vi "Add Pattern Part.vi"(4 "Suffix":string, 6 "Prefix":string, 8 "Modifier Token":T1, 9 "Regexp or Wildcard Token":T1, 10 "Name Token":T1, 11 "Pattern Parser In":T3) -> (0 "error out":errorcluster, 3 "Pattern Parser":T3)   [LabVIEW 2020, in "Stream.lvlib" / "URLPattern.lvclass"]
uses:
  URLPattern.lvclass
  Pattern Part Modifier.ctl
  Pattern Part Type.ctl
  Pattern Part.ctl
  Token Type.ctl
  Token.ctl
  Pattern Parser.ctl
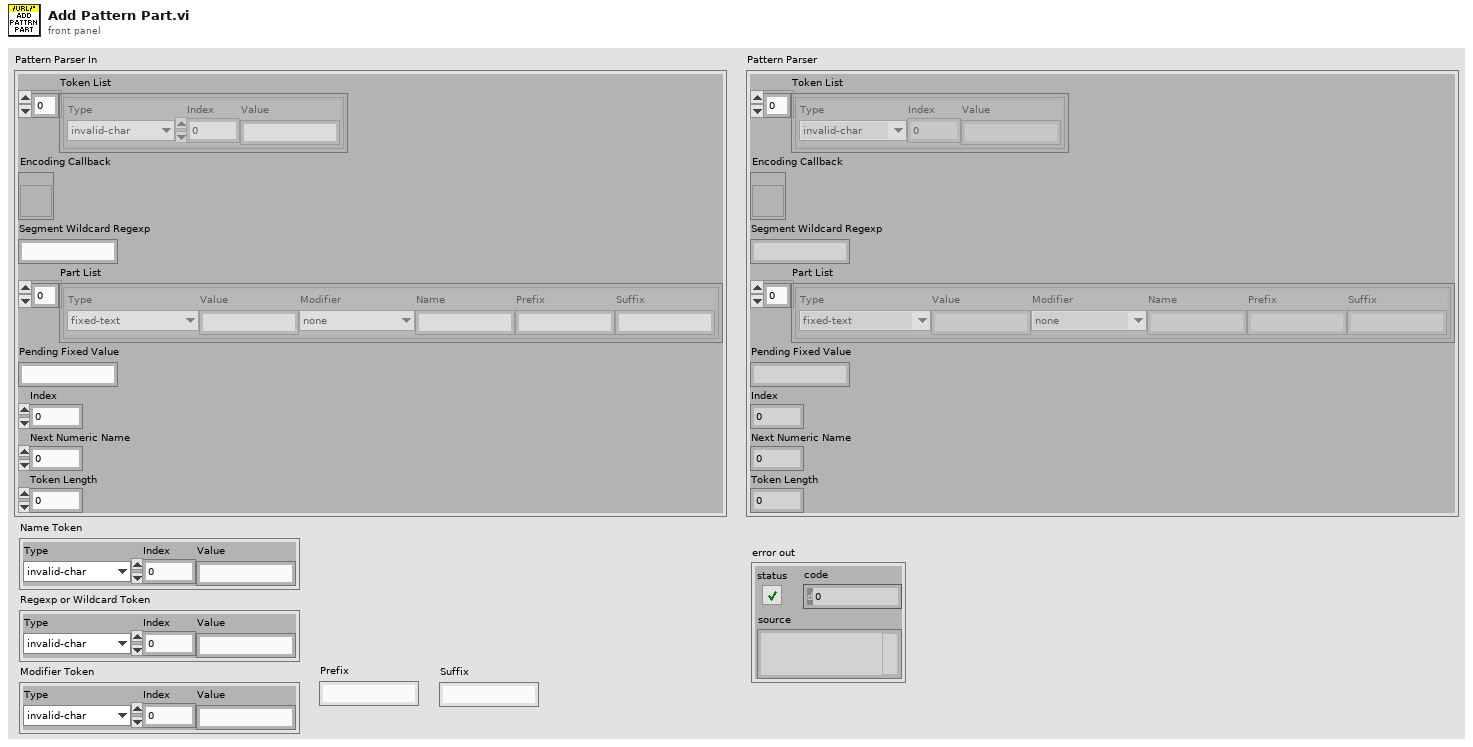
[diagram p1: front panel]
types:
  T1 = typedef "Stream.lvlib/URLPattern.lvclass/Token.ctl" = cluster{"Type":T2, "Index":i32, "Value":string}
  T2 = typedef "Stream.lvlib/URLPattern.lvclass/Token Type.ctl" = enum16{"invalid-char", "open", "close", "regexp", "name", "char", "escaped-char", "other-modifier", "asterisk", "end"}
  T3 = typedef "Stream.lvlib/URLPattern.lvclass/Pattern Parser.ctl" = cluster{"Token List":T1[], "Encoding Callback":refnum<vi>, "Segment Wildcard Regexp":string, "Part List":T4[], "Pending Fixed Value":string, "Index":i32, "Next Numeric Name":i32, "Token Length":i32}
  T4 = typedef "Stream.lvlib/URLPattern.lvclass/Pattern Part.ctl" = cluster{"Type":T5, "Value":string, "Modifier":T6, "Name":string, "Prefix":string, "Suffix":string}
  T5 = typedef "Stream.lvlib/URLPattern.lvclass/Pattern Part Type.ctl" = enum16{"fixed-text", "regexp", "segment-wildcard", "full-wildcard"}
  T6 = typedef "Stream.lvlib/URLPattern.lvclass/Pattern Part Modifier.ctl" = enum16{"none", "optional", "zero-or-more", "one-or-more"}
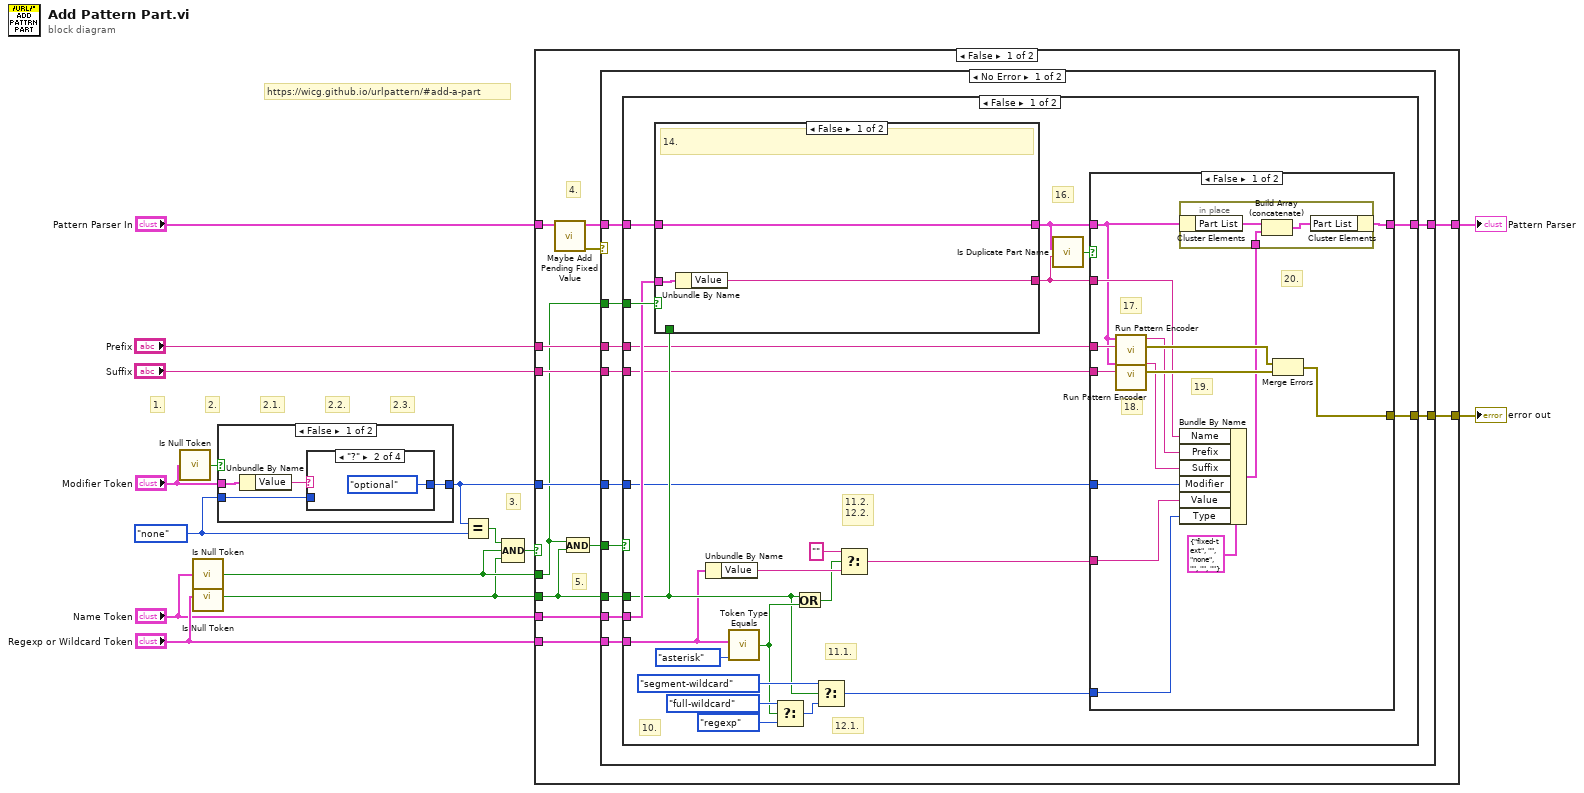
[diagram p0: block diagram]
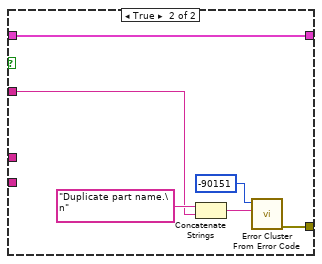
[diagram p2: hidden frame]
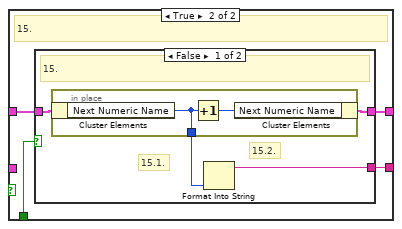
[diagram p3: hidden frame]
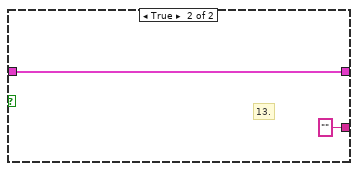
[diagram p4: hidden frame]
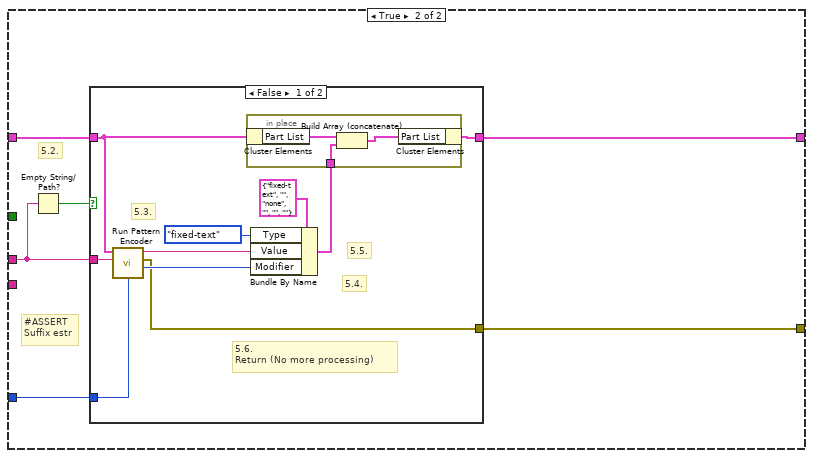
[diagram p5: hidden frame]
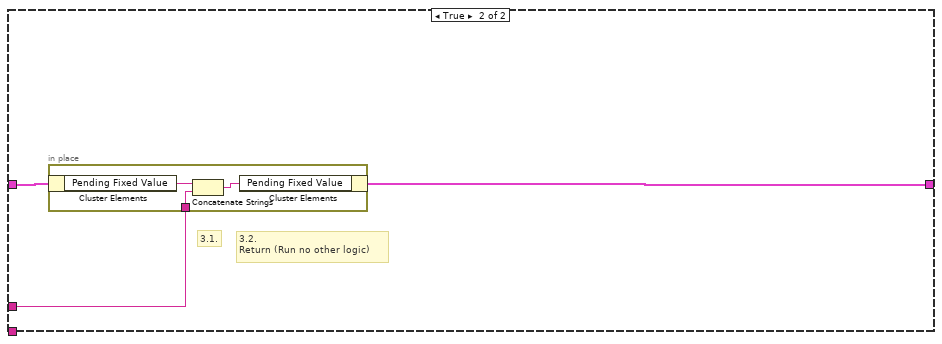
[diagram p8: hidden frame]
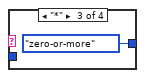
[diagram p10: hidden frame]
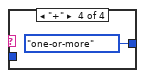
[diagram p11: hidden frame]
diagram:
  w7 = Pattern_Part_Modifier."none" ("Pattern Part Modifier")
  # "3."
  # "2.3."
  # "2.2."
  # "2.1."
  # "2."
  # "1."
  # "https://wicg.github.io/urlpattern/#add-a-part"
  n1 = call "Is Null Token.vi"("Token"="Modifier Token") -> ("Null Token"=w15:bool)
  n2 = call "Is Null Token.vi"("Token"="Name Token") -> ("Null Token"=w5:bool)
  n3 = call "Is Null Token.vi"("Token"="Regexp or Wildcard Token") -> ("Null Token"=w4:bool)
  n4 = case shown="False" w15 {
    tunnel: "Modifier Token" -> [w19 _]
    tunnel: [w17 w24] -> w6
    tunnel: w7 -> [w16 w24]
    frame False {
      n5 = Unbundle By Name(w19) -> ("Value"=w18:string)
      n6 = case shown="\"?\"" w18 {
        tunnel: [w20 Pattern_Part_Modifier."optional" ("Pattern Part Modifier") Pattern_Part_Modifier."zero-or-more" ("Pattern Part Modifier") Pattern_Part_Modifier."one-or-more" ("Pattern Part Modifier")] -> w17
        tunnel: w16 -> [w20 _ _ _]
        frame Default {
        }
        frame "?" {
        }
        frame "*" {
        }
        frame "+" {
        }
      }
    }
    frame True {
    }
  }
  n7 = Equal?(x=w6, y=w7) -> (x = y?=w13:bool)
  n8 = Compound Arithmetic op=AND(w13, w5, w4) -> (w12:bool)
  n9 = case shown="False" w12 {
    tunnel: "Pattern Parser In" -> [w37 w135]
    tunnel: "Prefix" -> [w33 w134]
    tunnel: [w32 w133] -> w9
    tunnel: "Suffix" -> [w35 _]
    tunnel: w6 -> [w31 _]
    tunnel: w5 -> [w28 _]
    tunnel: w4 -> [w29 _]
    tunnel: "Regexp or Wildcard Token" -> [w30 _]
    tunnel: "Name Token" -> [w27 _]
    tunnel: [w26 _] -> w1
    frame False {
      # "5."
      # "4."
      n10 = call "Maybe Add Pending Fixed Value.vi"("Pattern Parser In"=w37) -> ("error out"=w25:errorcluster, "Pattern Parser"=w36:T3)  [unwired: 9 in]
      n11 = And(x=w28, y=w29) -> (x .and. y?=w34:bool)
      n12 = case shown="No Error" w25 {
        selector: w25 -> [_ w132]
        tunnel: w36 -> [w48 w131]
        tunnel: w35 -> [w47 _]
        tunnel: w34 -> [w46 _]
        tunnel: w33 -> [w45 _]
        tunnel: [w44 w131] -> w32
        tunnel: w31 -> [w43 _]
        tunnel: w30 -> [w42 _]
        tunnel: w29 -> [w41 _]
        tunnel: w28 -> [w40 _]
        tunnel: w27 -> [w39 _]
        tunnel: [w38 w132] -> w26
        frame No Error {
          n13 = case shown="False" w46 {
            tunnel: w48 -> [w59 w116]
            tunnel: w47 -> [w52 _]
            tunnel: w45 -> [w53 w114]
            tunnel: [w54 w115] -> w44
            tunnel: w43 -> [w50 w113]
            tunnel: w42 -> [w60 _]
            tunnel: w41 -> [w61 _]
            tunnel: w40 -> [w63 _]
            tunnel: w39 -> [w62 _]
            tunnel: [w55 w112] -> w38
            frame False {
              # "16."
              # "11.2.\n12.2."
              # "10."
              # "12.1."
              # "11.1."
              n14 = case shown="False" w63 {
                tunnel: w62 -> [w99 _]
                tunnel: [w98 w101] -> w56
                tunnel: w61 -> [_ w103]
                tunnel: w59 -> [w97 w102]
                tunnel: [w97 w100] -> w58
                frame False {
                  # "14."
                  n15 = Unbundle By Name(w99) -> ("Value"=w98:string)
                }
                frame True {
                  # "15."
                  n16 = case shown="False" w103 {
                    tunnel: w102 -> [w107 w110]
                    tunnel: [w105 ""] -> w101
                    tunnel: [w104 w110] -> w100
                    frame False {
                      # "15.2."
                      # "15.1."
                      # "15."
                      n17 = in-place {
                        in-place-border: [w108] -> w106
                        n18 = in-place-cluster #1(w107) -> ("Next Numeric Name"=w108:i32)
                        n19 = Increment(x=w108) -> (x+1=w109:i32)
                        n20 = in-place-cluster #1("Next Numeric Name"=w109) -> (w104:T3)
                      }
                      n21 = Format Into String(w106) -> (resulting string=w105:string)  [unwired: 3 in, 1 out]
                    }
                    frame True {
                      # "13."
                    }
                  }
                }
              }
              n22 = Unbundle By Name(w60) -> ("Value"=w67:string)
              n23 = call "Token Type Equals.vi"("Type"=Token_Type."asterisk", "Token"=w60) -> ("Type Equals?"=w68:bool)  [unwired: 2 in]
              n24 = Select(t=Pattern_Part_Type."full-wildcard" ("Pattern Part Type"), s=w68, f=Pattern_Part_Type."regexp" ("Pattern Part Type")) -> (s? t:f=w64:T5)
              n25 = Or(x=w61, y=w68) -> (x .or. y?=w66:bool)
              n26 = Select(t=Pattern_Part_Type."segment-wildcard" ("Pattern Part Type"), s=w61, f=w64) -> (s? t:f=w51:T5)
              n27 = Select(t="" ("f"), s=w66, f=w67) -> (s? t:f=w49:string)
              n28 = call "Is Duplicate Part Name.vi"("Name"=w56, "Pattern Parser"=w58) -> ("Duplicate Name?"=w57:bool)  [unwired: 2 in]
              n29 = case shown="False" w57 {
                tunnel: w58 -> [w78 w91]
                tunnel: w56 -> [w79 w93]
                tunnel: [w73 w92] -> w55
                tunnel: [w76 w91] -> w54
                tunnel: w53 -> [w84 _]
                tunnel: w52 -> [w85 _]
                tunnel: w51 -> [w82 _]
                tunnel: w50 -> [w80 _]
                tunnel: w49 -> [w81 _]
                frame False {
                  # "20."
                  # "19."
                  # "18."
                  # "17."
                  n30 = call "Run Pattern Encoder.vi"("Input"=w84, "Pattern Parser"=w78) -> ("error out"=w86:errorcluster, "Encoded"=w74:string)  [unwired: 8 in]
                  n31 = call "Run Pattern Encoder.vi"("Input"=w85, "Pattern Parser"=w78) -> ("error out"=w87:errorcluster, "Encoded"=w75:string)  [unwired: 8 in]
                  n32 = Bundle By Name(cluster=T4 {"Type"=enum."fixed-text", "Value"="", "Modifier"=enum."none", "Name"="", "Prefix"="", "Suffix"=""} ("Pattern Part"), "Name"=w79, "Prefix"=w74, "Suffix"=w75, "Modifier"=w80, "Value"=w81, "Type"=w82) -> (w77:T4)
                  n33 = in-place {
                    in-place-border: w77 -> [w88]
                    n34 = in-place-cluster #2(w78) -> ("Part List"=w90:T4[])
                    n35 = Build Array (concatenate)(w90, w88) -> (w89:T4[])
                    n36 = in-place-cluster #2("Part List"=w89) -> (w76:T3)
                  }
                  n37 = Merge Errors(w86, w87) -> (w73:errorcluster)
                }
                frame True {
                  n38 = Concatenate Strings("Duplicate part name.\n" ("error message (\"\")"), w93) -> (w94:string)
                  n39 = call <vilib>:"Error Cluster From Error Code.vi"("error message (\"\")"=w94, "error code (0)"=-90151) -> ("error out"=w92:errorcluster)  [unwired: 7 in]
                }
              }
            }
            frame True {
              # "5.2."
              # "#ASSERT\nSuffix estr"
              n40 = Empty String/Path?(string/path=w114) -> (empty?=w117:bool)
              n41 = case shown="False" w117 {
                tunnel: w116 -> [w122 w130]
                tunnel: [w120 w130] -> w115
                tunnel: w114 -> [w126 _]
                tunnel: w113 -> [w123 _]
                tunnel: [w118 _] -> w112
                frame False {
                  # "5.6.\nReturn (No more processing)"
                  # "5.5."
                  # "5.4."
                  # "5.3."
                  n42 = call "Run Pattern Encoder.vi"("Input"=w126, "Pattern Parser"=w122) -> ("error out"=w118:errorcluster, "Encoded"=w119:string)  [unwired: 8 in]
                  n43 = Bundle By Name(cluster=T4 {"Type"=enum."fixed-text", "Value"="", "Modifier"=enum."none", "Name"="", "Prefix"="", "Suffix"=""} ("Pattern Part"), "Type"=Pattern_Part_Type."fixed-text", "Value"=w119, "Modifier"=w123) -> (w121:T4)
                  n44 = in-place {
                    in-place-border: w121 -> [w127]
                    n45 = in-place-cluster #3(w122) -> ("Part List"=w129:T4[])
                    n46 = Build Array (concatenate)(w129, w127) -> (w128:T4[])
                    n47 = in-place-cluster #3("Part List"=w128) -> (w120:T3)
                  }
                }
                frame True {
                  # "5.2.\nReturn (No other processing)"
                }
              }
            }
          }
        }
        frame Error {
        }
      }
    }
    frame True {
      # "3.2.\nReturn (Run no other logic)"
      # "3.1."
      n48 = in-place {
        in-place-border: w134 -> [w137]
        n49 = in-place-cluster #4(w135) -> ("Pending Fixed Value"=w138:string)
        n50 = Concatenate Strings(w138, w137) -> (w136:string)
        n51 = in-place-cluster #4("Pending Fixed Value"=w136) -> (w133:T3)
      }
    }
  }
  "Pattern Parser" <- w9
  "error out" <- w1
